vi "Initialize.vi"(8 "error in (no error)":errorcluster, 9 "modes of operations":i8(ring)=1 items=["Profile Position Mode"=1, "Profile Velocity Mode"=3, "Homing Mode"=6, "Interpolated Position Mode"=7, "Position Mode"=-1, "Velocity Mode"=-2, "Current Mode"=-3, "Master Encoder Mode"=-5, "Step Direction Mode"=-6], 10 "nodeId":u16=1, 11 "communication settings in":T1={"deviceName"="EPOS2", "protocolStackName"="MAXON SERIAL V2", "interfaceName"="USB", "portName"="USB0", "baudrate"=1000000, "timeout"=100}) -> (0 "error out":errorcluster, 3 "axis out":cluster{"keyHandle":u32, "nodeId":u16}={"keyHandle"=0, "nodeId"=1})   [LabVIEW 2018]
doc: "<B>Initialize</B> opens the port for sending and receiving commands. This function opens interfaces with the RS232 or USB and with CANopen boards.\nFor exact names use the functions <B>VCS Get Device Name Selection</B>, <B>VCS Get Protocol Stack Name Selection</B>, <B>VCS Get Interface Name Selection</B>, <B>VCS Get Port Name Selection</B> and <B>VCS Get Baudrate Selection</B>.\nThe function sets a new operational mode and clears all errors."
panel:
  # "(c) 2007 - 2017 maxon motor ag.  ALL RIGHTS RESERVED."
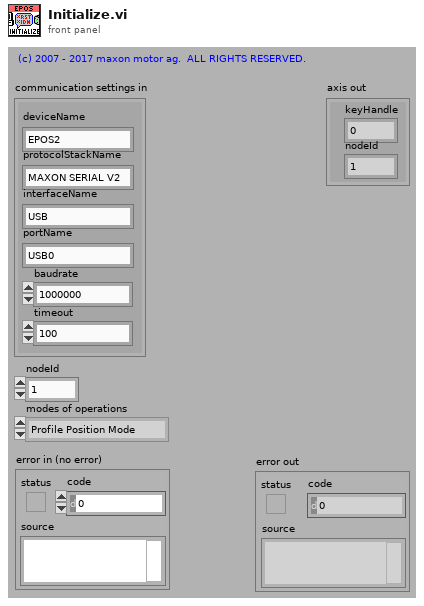
[diagram p1: front panel]
types:
  T1 = cluster{"deviceName":string, "protocolStackName":string, "interfaceName":string, "portName":string, "baudrate":u32, "timeout":u32}
  T2 = cluster{"deviceName":string, "protocolStackName":string, "interfaceName":string, "portName":string}
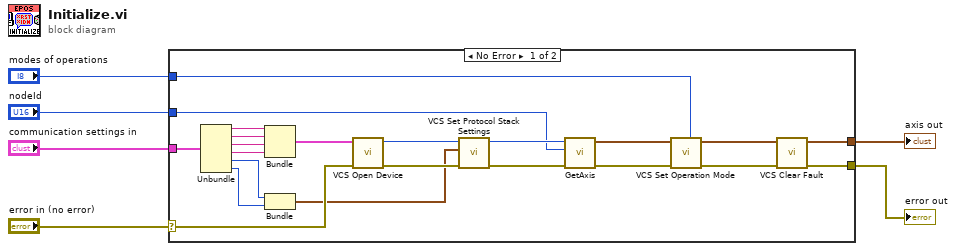
[diagram p0: block diagram]
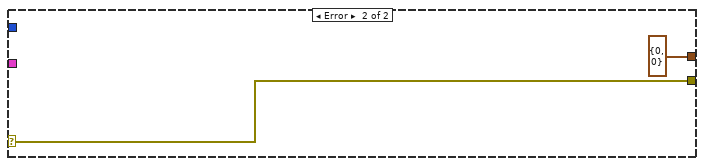
[diagram p2: hidden frame]
diagram:
  n1 = case shown="No Error" "error in (no error)" {
    selector: "error in (no error)" -> [w28 w30]
    tunnel: [w22 w30] -> w5
    tunnel: "communication settings in" -> [w15 _]
    tunnel: "nodeId" -> [w20 _]
    tunnel: "modes of operations" -> [w19 _]
    tunnel: [w16 cluster{"keyHandle":u32, "nodeId":u16} {"keyHandle"=0, "nodeId"=0} ("axis out")] -> w1
    frame No Error {
      n2 = Unbundle(w15) -> ("deviceName"=w11:string, "protocolStackName"=w10:string, "interfaceName"=w9:string, "portName"=w8:string, "baudrate"=w13:u32, "timeout"=w14:u32)
      n3 = Bundle("deviceName"=w11, "protocolStackName"=w10, "interfaceName"=w9, "portName"=w8) -> (w7:T2)  [unwired: 1 in]
      n4 = Bundle("baudrate"=w13, "timeout"=w14) -> (w12:cluster{"baudrate":u32, "timeout":u32})  [unwired: 1 in]
      n5 = call "VCS Open Device.vi"("error in (no error)"=w28, "device in"=w7) -> ("error out"=w27:errorcluster, "keyHandle out"=w26:u32)  [unwired: 8 in]
      n6 = call "VCS Set Protocol Stack Settings.vi"("error in (no error)"=w27, "settings"=w12, "keyHandle in"=w26) -> ("error out"=w25:errorcluster, "keyHandle out"=w21:u32)  [unwired: 7 in]
      n7 = call "GetAxis.vi"("error in (no error)"=w25, "nodeId"=w20, "keyHandle in"=w21) -> ("error out"=w24:errorcluster, "axis out"=w18:cluster{"keyHandle":u32, "nodeId":u16})  [unwired: 7 in]
      n8 = call "VCS Set Operation Mode.vi"("error in (no error)"=w24, "modes of operations"=w19, "axis in"=w18) -> ("error out"=w23:errorcluster, "axis out"=w17:cluster{"keyHandle":u32, "nodeId":u16})  [unwired: 7 in]
      n9 = call "VCS Clear Fault.vi"("error in (no error)"=w23, "axis in"=w17) -> ("error out"=w22:errorcluster, "axis out"=w16:cluster{"keyHandle":u32, "nodeId":u16})  [unwired: 8 in]
    }
    frame Error {
    }
  }
  "error out" <- w5
  "axis out" <- w1
